vi "USB_Identification.vi"() -> ()   [LabVIEW 2019]
panel:
  out "error out":errorcluster
  out "Interface Information:Interface Description":string
  in  "VISA resource name":refnum<visa-resource-name>
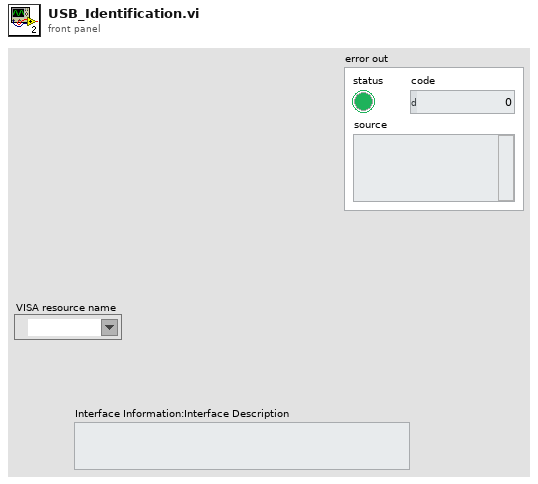
[diagram p1: front panel]
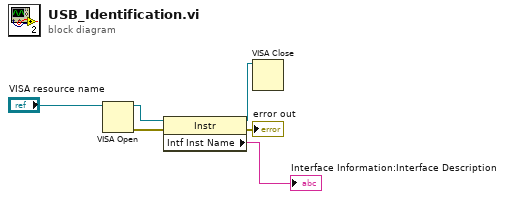
[diagram p0: block diagram]
diagram:
  n1 = VISA Open(VISA resource name="VISA resource name") -> (VISA resource name=w5:refnum<visa-resource-name>, error out=w6:errorcluster)  [unwired: 4 in]
  n2 = property class="Instr"(reference=w5, error in=w6) -> (reference out=w4:refnum<visa-resource-name>, error out=→"error out":errorcluster, "Intf Inst Name"=→"Interface Information:Interface Description":string)
  n3 = VISA Close(VISA resource name=w4) -> ()  [unwired: 1 in, 1 out]
